vi "ReferencedVariables_DeleteReferenceVariable_6x8x6.vi"(0 "reference in":refnum<class>, 5 "error in (no error)":errorcluster) -> (14 "reference out":refnum<class>, 16 "VariableReference":T1, 19 "error out":errorcluster)   [LabVIEW 2016]
doc: "This VI deletes a DVR reference variable."
uses:
  <resource>/Framework/Providers/Open_GDS/ClassProviders/DesignPatterns/ReferencedVariables/ReferencedVariables_SubVIs/ReferencedVariable.ctl
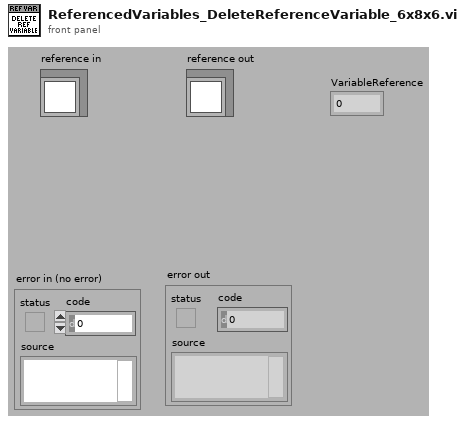
[diagram p1: front panel]
types:
  T1 = typedef "ReferencedVariable.ctl" = i32
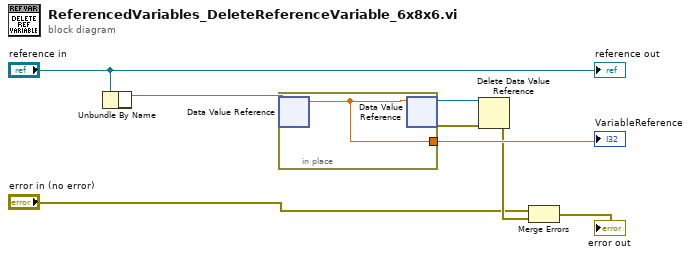
[diagram p0: block diagram]
diagram:
  n1 = Unbundle By Name("reference in") -> (w7)
  n2 = in-place {
    in-place-border: [w9] -> w6
    n3 = in-place-dvr #1(w7) -> (w9:dbl)  [unwired: 1 out]
    n4 = in-place-dvr #1(w9) -> (w5:refnum<data-value>, w4:errorcluster)
  }
  "VariableReference" <- w6
  n5 = Delete Data Value Reference(data value reference=w5, error in=w4) -> (error out=w3:errorcluster)  [unwired: 1 out]
  n6 = Merge Errors("error in (no error)", w3) -> (→"error out":errorcluster)
  "reference out" <- "reference in"
